vi "Load config.vi"(8 "error in":errorcluster, 11 "INI data":T1) -> (0 "error out":errorcluster, 3 "INI data out":T1)   [LabVIEW 2014]
uses:
  Controls/INI config.ctl
  <vilib>/Utility/config.llb/Read Key (String).vi
  <vilib>/Utility/config.llb/NI_LVConfig.lvlib
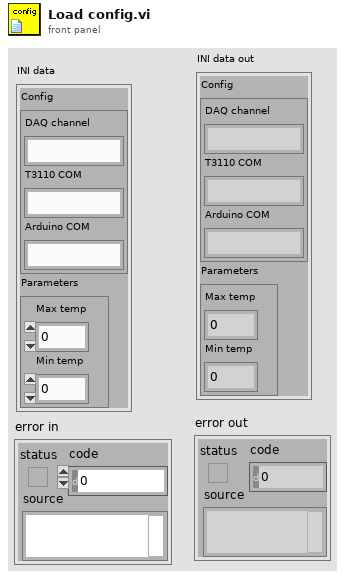
[diagram p1: front panel]
types:
  T1 = typedef "INI config.ctl" = cluster{"Config":cluster{"DAQ channel":string, "T3110 COM":string, "Arduino COM":string}, "Parameters":cluster{"Max temp":dbl, "Min temp":dbl}}
  T2 = typedef "NI_LVConfig.lvlib/Config Data RefNum.ctl" = refnum<k1>
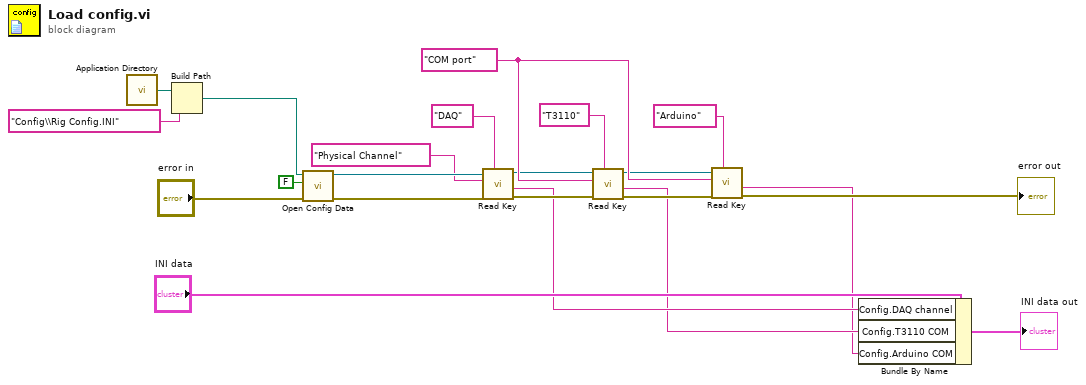
[diagram p0: block diagram]
diagram:
  w7 = "COM port" ("key")
  n1 = call <vilib>:"Application Directory.vi"() -> ("Application Directory"=w16:path)
  n2 = Build Path(base path=w16, name or relative path="Config\\Rig Config.INI") -> (appended path=w14:path)
  n3 = call <vilib>:"Open Config Data.vi"("error in (no error)"="error in", "create file if necessary (T)"=FALSE, "configuration file path"=w14) -> ("error out"=w19:errorcluster, "refnum"=w21:T2)  [unwired: 6 in, 1 out]
  n4 = call-poly <vilib>:"Read Key.vi"("section"="DAQ", "error in (no error)"=w19, "key"="Physical Channel", "refnum"=w21) -> ("error out"=w12:errorcluster, "value"=w6:string, "refnum out"=w2:T2)  [unwired: 4 in, 1 out]
  n5 = call-poly <vilib>:"Read Key.vi"("section"="T3110", "error in (no error)"=w12, "key"=w7, "refnum"=w2) -> ("error out"=w11:errorcluster, "value"=w5:string, "refnum out"=w1:T2)  [unwired: 4 in, 1 out]
  n6 = call-poly <vilib>:"Read Key.vi"("section"="Arduino", "error in (no error)"=w11, "key"=w7, "refnum"=w1) -> ("error out"=→"error out":errorcluster, "value"=w4:string)  [unwired: 4 in, 2 out]
  n7 = Bundle By Name(cluster="INI data", "Config.DAQ channel"=w6, "Config.T3110 COM"=w5, "Config.Arduino COM"=w4) -> (→"INI data out":T1)
